vi "notification log.vi"(1 "Notification":string, 2 "Clear Log":bool) -> (0 "Output Log":string[][](array[string]))   [LabVIEW 2015]
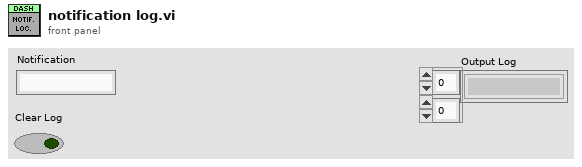
[diagram p1: front panel]
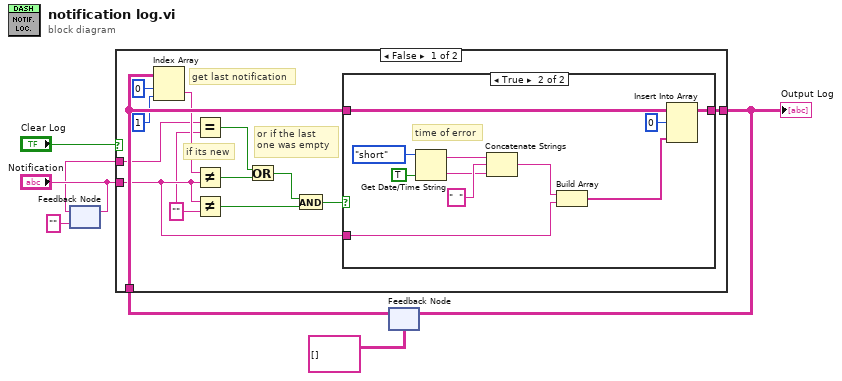
[diagram p0: block diagram]
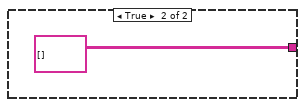
[diagram p3: hidden frame]
diagram:
  n1 = feedback #1("" ("Notification")) -> (w2:string)
  n2 = feedback-in #1("Notification") -> ()
  n3 = feedback #2(string[][] [] ("Output Log")) -> (w6:string[][])
  n4 = case shown="False" "Clear Log" {
    tunnel: w6 -> [w20 _]
    tunnel: [w15 string[][] [] ("Output Log")] -> w4
    tunnel: "Notification" -> [w14 _]
    tunnel: w2 -> [w11 _]
    frame False {
      w10 = "" ("y")
      # "or if the last\none was empty"
      # "if its new"
      # "get last notification"
      n5 = Index Array(array=w20, index (row)=0, index (col)=1 ("disabled index (col)")) -> (element=w17:string)
      n6 = Equal?(x=w11, y=w10) -> (x = y?=w9:bool)
      n7 = Not Equal?(x=w17, y=w14) -> (x != y?=w12:bool)
      n8 = Not Equal?(x=w14, y=w10) -> (x != y?=w13:bool)
      n9 = Or(x=w9, y=w12) -> (x .or. y?=w8:bool)
      n10 = And(x=w8, y=w13) -> (x .and. y?=w16:bool)
      n11 = case shown="True" w16 {
        tunnel: w20 -> [w21 w27]
        tunnel: [w21 w26] -> w15
        tunnel: w14 -> [_ w23]
        frame False {
        }
        frame True {
          # "time of error"
          n12 = Get Date/Time String(date format (0)=enum16{"short", "long", "abbreviated"}."short", want seconds? (F)=TRUE) -> (date string=w29:string, time string=w28:string)  [unwired: 1 in]
          n13 = Concatenate Strings(w29, "  " ("string"), w28) -> (w24:string)
          n14 = Build Array(w24, w23) -> (w22:string[])
          n15 = Insert Into Array(array=w27, index (row)=0, new element=w22) -> (w26:string[][])  [unwired: 1 in]
        }
      }
    }
    frame True {
    }
  }
  "Output Log" <- w4
  n16 = feedback-in #2(w4) -> ()
